vi "sensor cmd led pattern.vi"(7 "length":u8, 9 "pattern":string, 10 "interval":u8, 11 "device_handle":u32) -> (1 "pattern out":string, 2 "function return":i32, 3 "device_handle out":u32)   [LabVIEW 2019, in "apdm.lvlib"]
doc: "APDM_EXPORT int apdm_sensor_cmd_led_pattern(apdm_device_handle_t device_handle, uint8_t interval, uint8_t *pattern, uint8_t length);"
uses:
  apdm.lvlib
  Lee Lab/CP FES Walking 2018/Code/Working/LabVIEW/apdm.dll
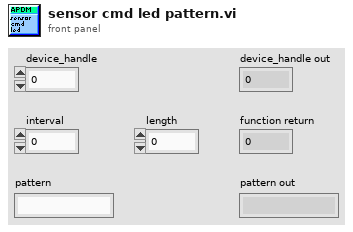
[diagram p1: front panel]
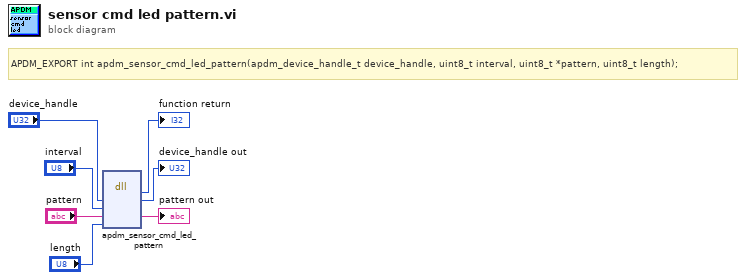
[diagram p0: block diagram]
diagram:
  # "APDM_EXPORT int apdm_sensor_cmd_led_pattern(apdm_device_handle_t device_handle, uint8_t interval, uint8_t *pattern, uint8_t length);"
  n1 = dll-call lib="C:/Users/jfalesi/Dropbox/Lee Lab/CP FES Walking 2018/Code/Working/LabVIEW/apdm.*" fn="apdm_sensor_cmd_led_pattern"("device_handle"="device_handle", "interval"="interval", "pattern"="pattern", "length"="length") -> (→"function return":i32, "device_handle"=→"device_handle out":u32, "pattern"=→"pattern out":string)  [unwired: 5 in, 2 out]
